vi "SQL_Select.vi"(6 "要读取的列名":string[](array[string]), 7 "表名":string, 8 "error in (no error)":errorcluster, 9 "查询语句":string, 10 "查询条件":bool=TRUE, 11 "connection reference":T1) -> (0 "error out":errorcluster, 2 "数据":string[][](array[string]), 3 "connection reference out":T1)   [LabVIEW 2018]
uses:
  <vilib>/addons/database/Connection.llb/Conn ObjectReference.ctl
  <vilib>/addons/database/Connection.llb/Conn Execute.vi
  <vilib>/addons/database/Recordset.llb/Rec Fetch Recordset Data (R).vi
  <vilib>/addons/database/Recordset.llb/Rec Destroy - Connection.vi
  <vilib>/addons/database/NI_Database_API.lvlib
panel:
  # "语法："
  # "SELECT 列名称 FROM 表名称"
  # "SELECT * FROM 表名称"
  # "例：where a='1'"
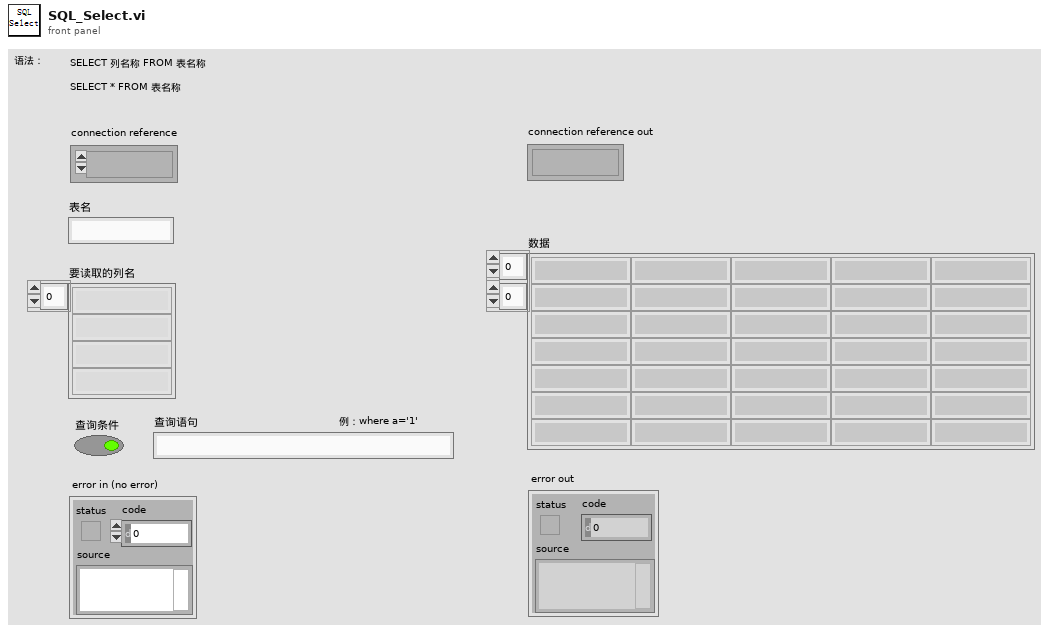
[diagram p1: front panel]
types:
  T1 = typedef "NI_Database_API.lvlib/Conn ObjectReference.ctl" = refnum<k1>
  T2 = typedef "NI_Database_API.lvlib/Rec ObjectReference.ctl" = refnum<k1>
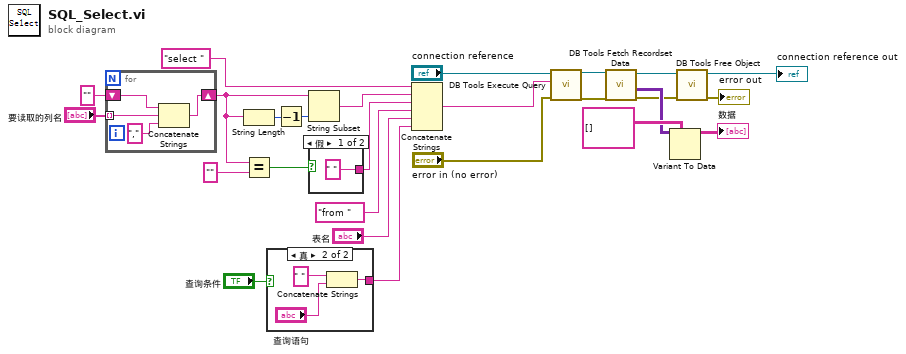
[diagram p0: block diagram]
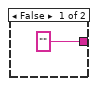
[diagram p2: hidden frame]
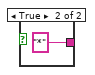
[diagram p3: hidden frame]
diagram:
  n1 = for {
    tunnel: "要读取的列名" -> [w30] mode=indexing
    shift-right: [w29] -> w18
    shift-left: "" -> [w27]
    n2 = Concatenate Strings(w27, w30, "," ("字符串")) -> (w29:string)
  }
  n3 = String Length(string=w18) -> (length=w17:i32)
  n4 = Equal?(x=w18, y="") -> (x = y?=w22:bool)
  n5 = case shown="真" "查询条件" {
    tunnel: ["" w34] -> w13
    frame False {
    }
    frame True {
      n6 = Concatenate Strings(" ", "查询语句") -> (w34:string)
    }
  }
  n7 = Decrement(x=w17) -> (x-1=w15:i32)
  n8 = String Subset(string=w18, length (rest)=w15) -> (substring=w16:string)  [unwired: 1 in]
  n9 = case shown="假" w22 {
    tunnel: [" " ("y") "*" ("y")] -> w21
    frame False {
    }
    frame True {
    }
  }
  n10 = Concatenate Strings("select ", w16, w21, "from ", "表名", w13) -> (w3:string)
  n11 = call-poly <vilib>:"DB Tools Execute Query.vi"("error in (no error)"="error in (no error)", "SQL query"=w3, "connection reference"="connection reference") -> ("error out"=w5:errorcluster, "recordset reference"=w4:T2)  [unwired: 5 in]
  n12 = call-poly <vilib>:"DB Tools Fetch Recordset Data.vi"("error in (no error)"=w5, "recordset reference"=w4) -> ("error out"=w9:errorcluster, "recordset data"=w10:variant[][], "recordset reference out"=w8:T2)  [unwired: 3 in]
  n13 = Variant To Data(type=string[][] [], Variant=w10) -> (data=→"数据":string[][])  [unwired: 1 in, 1 out]
  n14 = call-poly <vilib>:"DB Tools Free Object.vi"("error in (no error)"=w9, "recordset reference"=w8) -> ("error out"=→"error out":errorcluster, "connection reference"=→"connection reference out":T1)  [unwired: 8 in]
